vi "Set Front Panel Custom Image Size Cluster Control.vi"(8 "error in (no error)":errorcluster, 10 "Init":bool, 11 "Imaging Parameter":refnum<vi>) -> (0 "error IO":errorcluster)   [LabVIEW 2018]
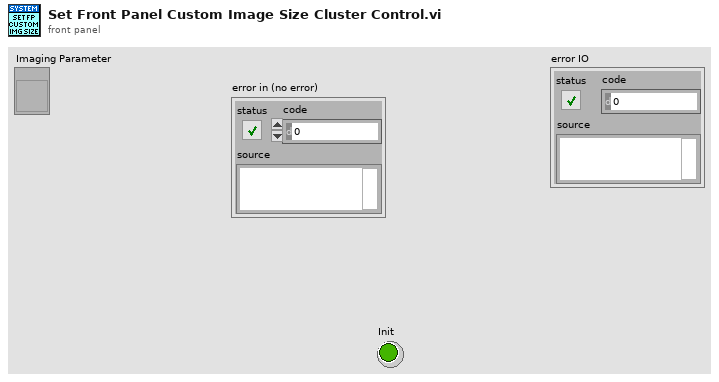
[diagram p1: front panel]
types:
  T1 = enum8{"Enabled", "Disabled", "Disabled and Grayed Out"}
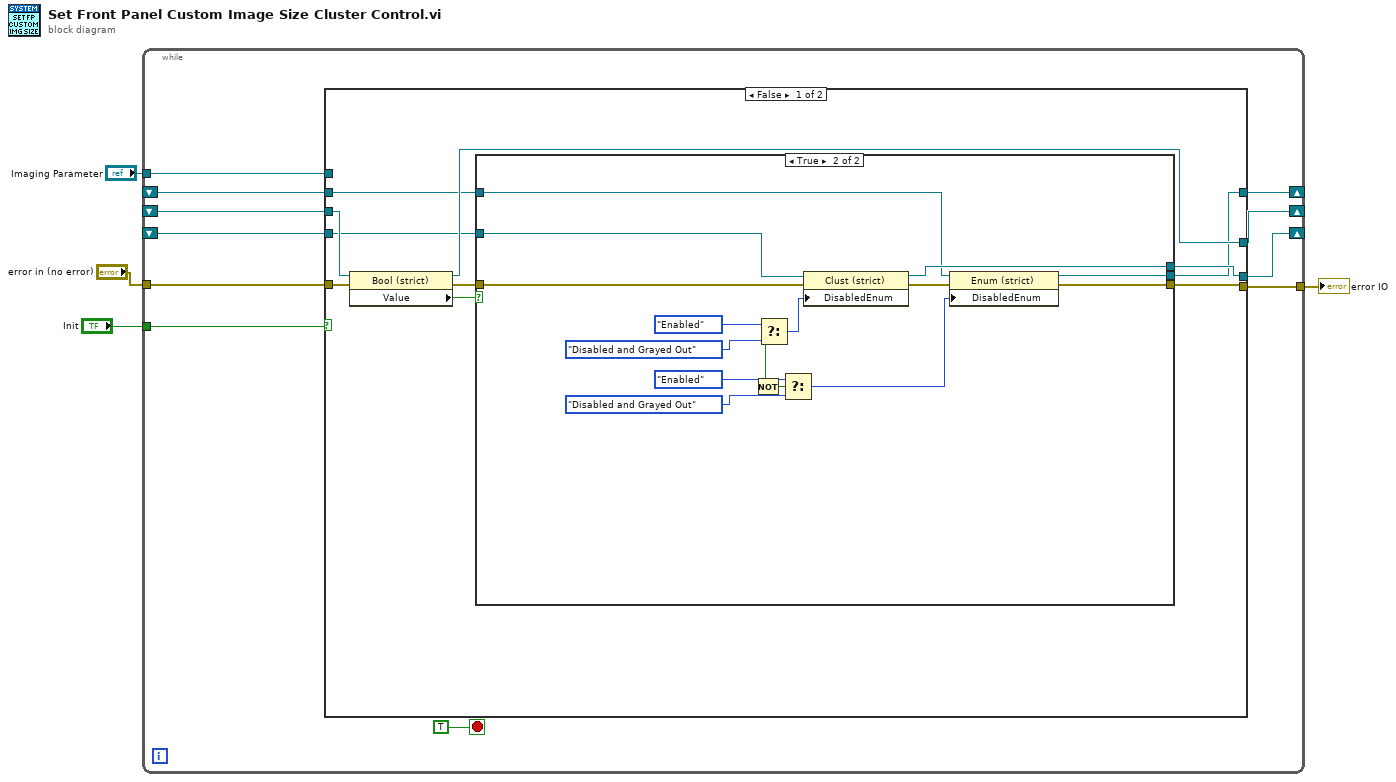
[diagram p0: block diagram]
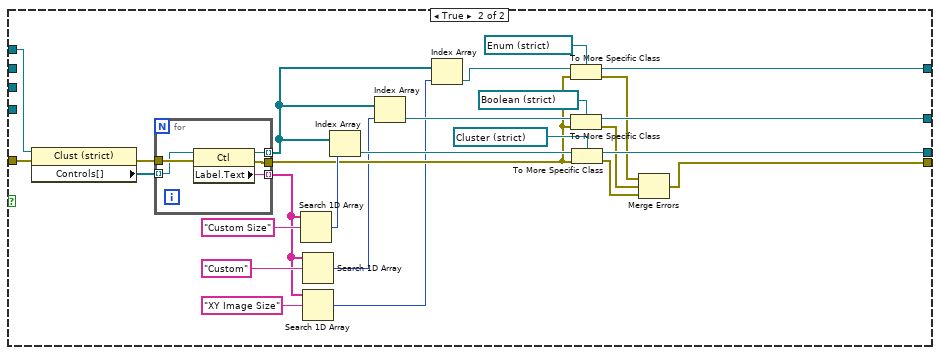
[diagram p3: hidden frame]
diagram:
  n1 = while {
    tunnel: "Imaging Parameter" -> [w15]
    tunnel: [w12] -> w3
    tunnel: "error in (no error)" -> [w11]
    shift-right: [w13] -> _
    shift-left: _ -> [w10]
    tunnel: "Init" -> [w9]
    shift-right: [w8] -> _
    shift-left: _ -> [w7]
    shift-right: [w6] -> _
    shift-left: _ -> [w5]
    stop <- TRUE stop-if-true
    n2 = case shown="False" w9 {
      tunnel: w15 -> [_ w66]
      tunnel: [w22 w56] -> w13
      tunnel: [w19 w53] -> w12
      tunnel: w11 -> [w25 w63]
      tunnel: w10 -> [w20 _]
      tunnel: [w21 w57] -> w8
      tunnel: w7 -> [w23 _]
      tunnel: [w17 w48] -> w6
      tunnel: w5 -> [w18 _]
      frame False {
        n3 = property class="Bool (strict)"(reference=w23, error in=w25) -> (reference out=w21:refnum<vi>, error out=w24:errorcluster, "Value"=w16:bool)
        n4 = case shown="True" w16 {
          tunnel: w24 -> [_ w40]
          tunnel: [_ w38] -> w22
          tunnel: w20 -> [_ w37]
          tunnel: [_ w33] -> w19
          tunnel: w18 -> [_ w32]
          tunnel: [_ w31] -> w17
          frame False {
          }
          frame True {
            n5 = Not() -> (x=w28:bool, .not. x?=w27:bool)
            n6 = Select(t=T1."Enabled" ("Disabled"), s=w28, f=T1."Disabled and Grayed Out" ("Disabled")) -> (s? t:f=w34:T1)
            n7 = Select(t=T1."Enabled" ("Disabled"), s=w27, f=T1."Disabled and Grayed Out" ("Disabled")) -> (s? t:f=w26:T1)
            n8 = property class="Clust (strict)"(reference=w37, error in=w40, "DisabledEnum"=w34) -> (reference out=w38:refnum<vi>, error out=w39:errorcluster)
            n9 = property class="Enum (strict)"(reference=w32, error in=w39, "DisabledEnum"=w26) -> (reference out=w31:refnum<vi>, error out=w33:errorcluster)
          }
        }
      }
      frame True {
        n10 = property class="Clust (strict)"(reference=w66, error in=w63) -> (error out=w64:errorcluster, "Controls[]"=w65:refnum<vi>[])  [unwired: 1 out]
        n11 = for {
          tunnel: w65 -> [w70] mode=indexing
          tunnel: w64 -> [w71]
          tunnel: [w69] -> w43 mode=indexing
          tunnel: [w68] -> w46 mode=indexing
          tunnel: [w67] -> w47
          n12 = property class="Ctl"(reference=w70, error in=w71) -> (reference out=w68:refnum<vi>, error out=w67:errorcluster, "Label.Text"=w69:string)
        }
        n13 = Search 1D Array(1D array=w43, element="Custom Size") -> (index of element=w60:i32)  [unwired: 1 in]
        n14 = Search 1D Array(1D array=w43, element="Custom") -> (index of element=w44:i32)  [unwired: 1 in]
        n15 = Search 1D Array(1D array=w43, element="XY Image Size") -> (index of element=w41:i32)  [unwired: 1 in]
        n16 = Index Array(array=w46, index=w60) -> (element=w61:refnum<vi>)
        n17 = Index Array(array=w46, index=w44) -> (element=w58:refnum<vi>)
        n18 = Index Array(array=w46, index=w41) -> (element=w45:refnum<vi>)
        n19 = To More Specific Class(target class=refnum<vi> refnum ("XY Image Size"), reference=w45, error in=w47) -> (specific class reference=w48:refnum<vi>, error out=w49:errorcluster)
        n20 = To More Specific Class(target class=refnum<vi> refnum ("Boolean"), reference=w58, error in=w47) -> (specific class reference=w57:refnum<vi>, error out=w54:errorcluster)
        n21 = To More Specific Class(target class=refnum<vi> refnum ("Custom Size"), reference=w61, error in=w47) -> (specific class reference=w56:refnum<vi>, error out=w55:errorcluster)
        n22 = Merge Errors(w49, w54, w55) -> (w53:errorcluster)
      }
    }
  }
  "error IO" <- w3
